vi "gyro.vi"   [LabVIEW 2012]
uses:
  Dropbox/FRC 2013/First 2013 Robot Project/Globals/Joysticks.vi
  Dropbox/FRC 2013/First 2013 Robot Project/Globals/Tachometer.vi
  <vilib>/addons/control/pid/pid.llb/PID (DBL).vi
  <vilib>/addons/control/pid/NI_PID_pid.lvlib
types:
  T1 = typedef "WPI_JoystickDevRef.ctl" = cluster{"Device":T2}
  T2 = typedef "WPI_JoystickDeviceEnum.ctl" = enum16{"USB 1", "USB 2", "USB 3", "USB 4", "Kinect 1", "Kinect 2"}
  T3 = cluster{"axis 1 (x)":dbl, "axis 2 (y)":dbl, "axis 3 (throttle)":dbl, "axis 4":dbl, "axis 5":dbl, "axis 6":dbl}
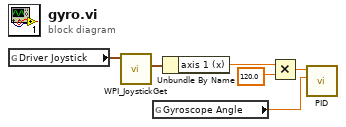
[diagram p0: block diagram]
diagram:
  n1 = global read "Joysticks.vi" "Driver Joystick"() -> (w6:T1)
  n2 = call <vilib>:"WPI_JoystickGet.vi"("JoystickDevRef"=w6) -> ("Axes"=w5:T3)  [unwired: 4 in, 2 out]
  n3 = global read "Tachometer.vi" "Gyroscope Angle"() -> (w1:dbl)
  n4 = Unbundle By Name(w5) -> ("axis 1 (x)"=w4:dbl)
  n5 = Multiply(x=w4, y=120.0) -> (x*y=w2:dbl)
  n6 = call-poly <vilib>:"PID.vi"("process variable"=w1, "setpoint"=w2) -> ()  [unwired: 8 in, 2 out]
